vi "Get Newest File Path.vi"(8 "error in (no error)":errorcluster, 10 "pattern":string="cal_*.csv", 11 "Path":path) -> (0 "error out":errorcluster, 2 "Newest File Name":string, 3 "Newest File Path":path)   [LabVIEW 2025, in "File System.lvlib"]
uses:
  File System.lvlib
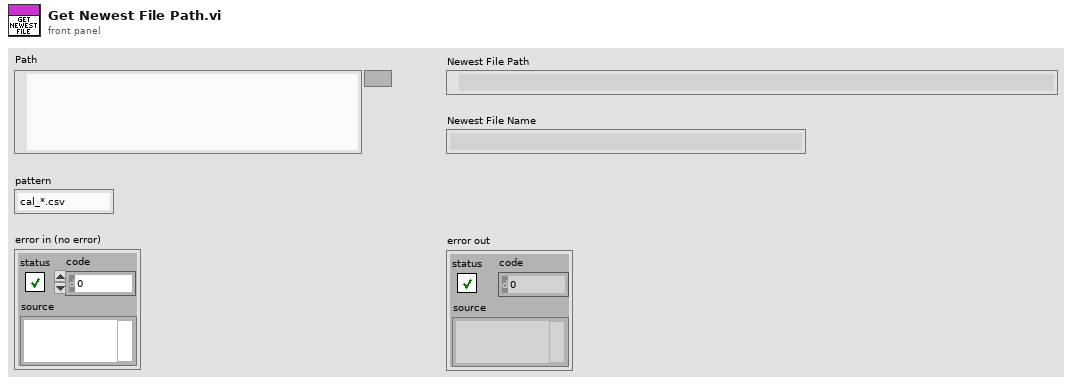
[diagram p1: front panel]
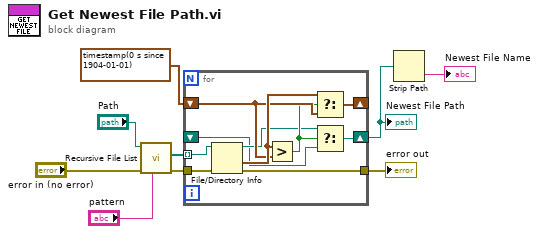
[diagram p0: block diagram]
diagram:
  n1 = call <vilib>:"Recursive File List.vi"("pattern"="pattern", "error in (no error)"="error in (no error)", "Folder Path"="Path") -> ("error out"=w6:errorcluster, "All Files in Dir"=w4:path[])  [unwired: 4 in, 3 out]
  n2 = for {
    tunnel: w4 -> [w19] mode=indexing
    tunnel: [w18] -> w1
    tunnel: w6 -> [w17]
    shift-right: [w10] -> w3
    shift-left: _ -> [w11]
    shift-right: [w14] -> _
    shift-left: timestamp(0 s since 1904-01-01) ("last mod") -> [w15]
    n3 = File/Directory Info(path=w19, error in=w17) -> (path out=w12:path, last mod=w16:timestamp, error out=w18:errorcluster)  [unwired: 4 out]
    n4 = Greater?(x=w16, y=w15) -> (0:w13:bool)
    n5 = Select(t=w16, s=w13, f=w15) -> (s? t:f=w14:timestamp)
    n6 = Select(t=w12, s=w13, f=w11) -> (s? t:f=w10:path)
  }
  "error out" <- w1
  "Newest File Path" <- w3
  n7 = Strip Path(path=w3) -> (name=→"Newest File Name":string)  [unwired: 1 out]
